vi "Random Generator.vi"() -> (2 "unsigned 16bit integer":u32, 3 "rnd.U32":u32)   [LabVIEW 2015]
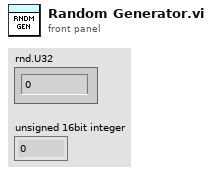
[diagram p1: front panel]
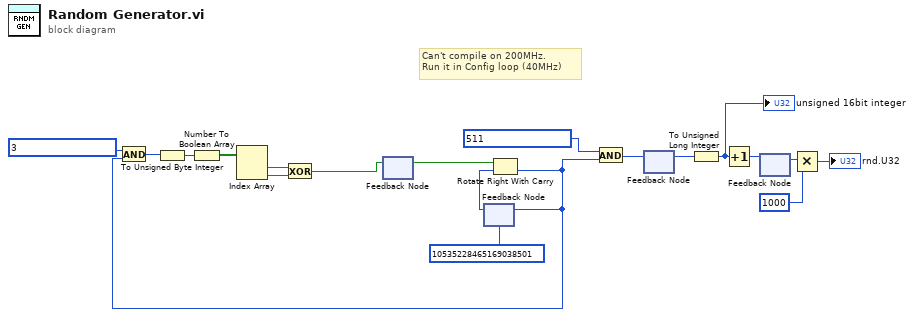
[diagram p0: block diagram]
diagram:
  # "Can't compile on 200MHz. \nRun it in Config loop (40MHz)"
  n1 = feedback #1() -> (w14:bool)  [unwired: 1 in]
  n2 = feedback #2(u64 10535228465169038501) -> (w6:u64)
  n3 = Rotate Right With Carry(2:w6, 3:w14) -> (0:w12:u64)  [unwired: 1 out]
  n4 = And(x=u64 3, y=w12) -> (x .and. y?=w7:u64)
  n5 = To Unsigned Byte Integer(number=w7) -> (unsigned 8bit integer=w8:u8)
  n6 = Number To Boolean Array(number=w8) -> (Boolean array=w11:bool[])
  n7 = Index Array(array=w11) -> (element #1=w9:bool, element #2=w10:bool)  [unwired: 2 in]
  n8 = Exclusive Or(1:w10, 2:w9) -> (0:w13:bool)
  n9 = feedback-in #1(w13) -> ()
  n10 = feedback-in #2(w12) -> ()
  n11 = And(x=u64 511, y=w12) -> (x .and. y?=w15:u64)
  n12 = feedback #3() -> (w16:u64)  [unwired: 1 in]
  n13 = feedback-in #3(w15) -> ()
  n14 = To Unsigned Long Integer(number=w16) -> (unsigned 32bit integer=w4:u32)
  "unsigned 16bit integer" <- w4
  n15 = Increment(x=w4) -> (x+1=w17:u32)
  n16 = feedback #4() -> (w18:u32)  [unwired: 1 in]
  n17 = feedback-in #4(w17) -> ()
  n18 = Multiply(x=w18, y=u32 1000) -> (x*y=→"rnd.U32":u32)
